vi "test Occurance Fired.vi"(8 "error in (no error)":errorcluster, 11 "TestCase in":refnum<class "Sync Tests.lvclass">) -> (0 "error out":errorcluster, 3 "TestCase out":refnum<class "Sync Tests.lvclass">)   [LabVIEW 2020, in "Sync Tests.lvclass"]
uses:
  Sync Tests.lvclass
  <vilib>/Utility/file.llb/Application Directory.vi
  <vilib>/Utility/libraryn.llb/Check if File or Folder Exists.vi
  <vilib>/addons/_JKI Toolkits/VI Tester/TestCase.llb/TestCase.lvclass
  C:/Program Files/National Instruments/LabVIEW 2020/vi.lib/addons/_JKI Toolkits/VI Tester/TestCase.llb/TestCase.lvclass
panel:
  out "return type":i32
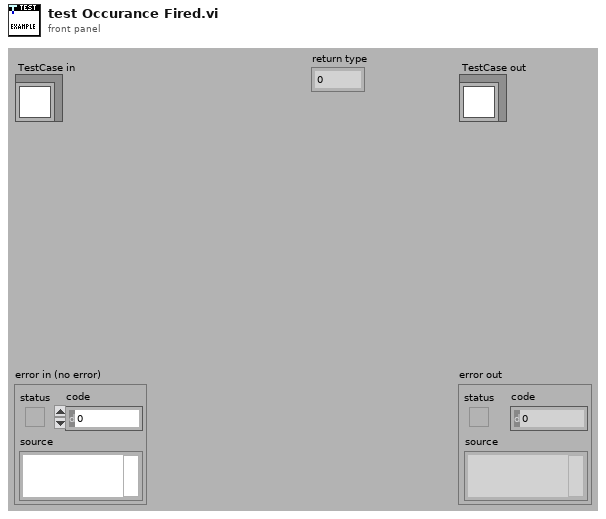
[diagram p1: front panel]
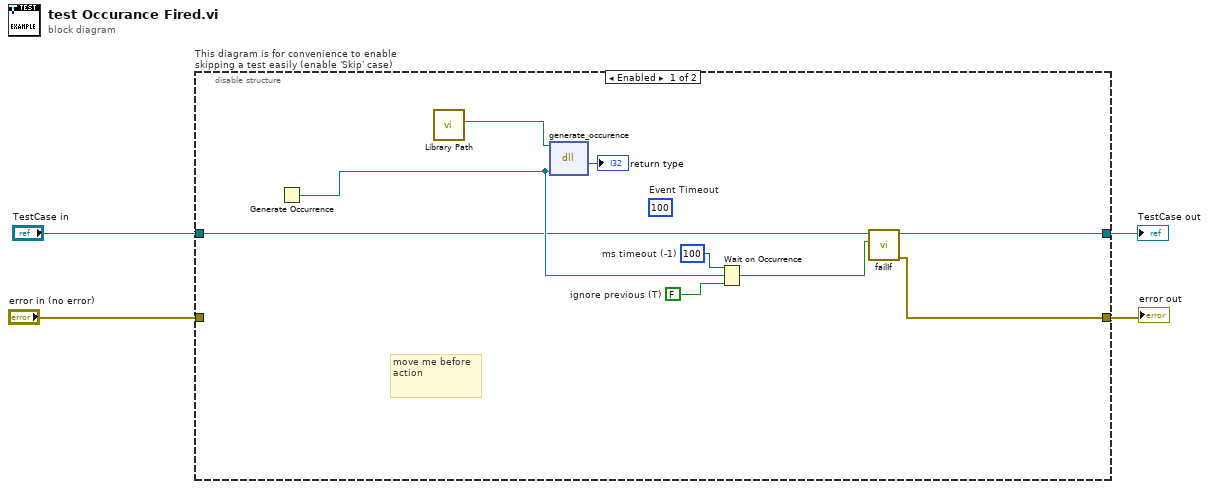
[diagram p0: block diagram]
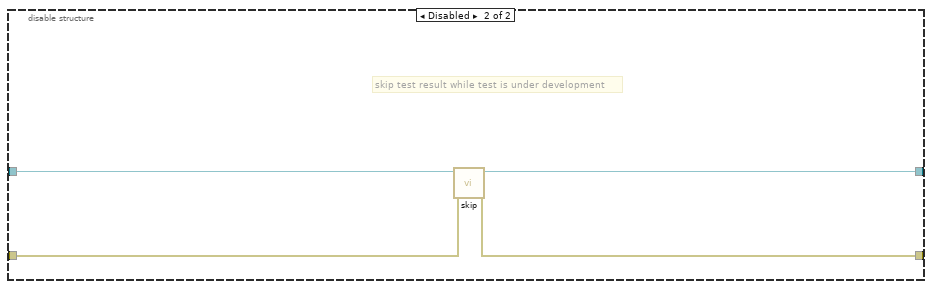
[diagram p2: hidden frame]
diagram:
  n1 = disable-structure "This diagram is for convenience to enable skipping a test easily (enable 'Skip' case)" shown="Enabled" {
    disable-tunnel: "TestCase in" -> [w8 w17]
    disable-tunnel: [w7 w15] -> w1
    disable-tunnel: [w6 w16] -> w3
    disable-tunnel: "error in (no error)" -> [_ w14]
    frame Enabled {
      w9 = FALSE  # ignore previous (T)
      w10 = 100  # ms timeout (-1)
      (unwired) 100  # Event Timeout
      # "move me before\naction"
      n2 = Generate Occurrence() -> (w11:refnum<k4>)
      n3 = call "Library Path.vi"() -> ("Library Path"=w13:path)  [unwired: 11 in]
      n4 = dll-call lib="C:/Users/JamesMcNally/Documents/RustInterop/Rust-LabVIEW-Interop/target/debug/labview_test_library.dll" fn="generate_occurence"(path in=w13, "occurence"=w11) -> ("return type"=→"return type":i32)  [unwired: 3 in, 2 out]
      n5 = Wait on Occurrence(1:w9, 2:w11, 3:w10) -> (0:w5:bool)
      n6 = call-dynamic "failIf.vi"("fail"=w5, "TestCase in"=w8) -> ("error out"=w6:errorcluster, "TestCase out"=w7:refnum<class "Sync Tests.lvclass">)  [unwired: 8 in]
    }
    frame Disabled {
      # "skip test result while test is under development"
      n7 = call <vilib>:"skip.vi"("error in (no error)"=w14, "TestCase in"=w17) -> ("error out"=w16:errorcluster, "TestCase out"=w15:refnum<class "Sync Tests.lvclass">)  [unwired: 8 in]
    }
  }
  "error out" <- w3
  "TestCase out" <- w1
